vi "Build Filter Command.vi"(8 "error in (no error)":errorcluster, 11 "Filter in":refnum<class "Filter.lvclass">) -> (0 "error out":errorcluster, 2 "Command Words":u16[](array[numeric]) format="%04x")   [LabVIEW 2020, in "BCI-1553 API.lvlib" / "Filter.lvclass"]
doc: "<DO NOT CALL>\n\nThis method is leveraged by the Bus Monitor to produce the raw configuration values for setting up a filter in hardware."
uses:
  Filter.lvclass
  Frames & Messages/TypeDefs/Command Type.ctl
  Filter.lvclass/Filter.ctl
  BCI-1553 API.lvlib
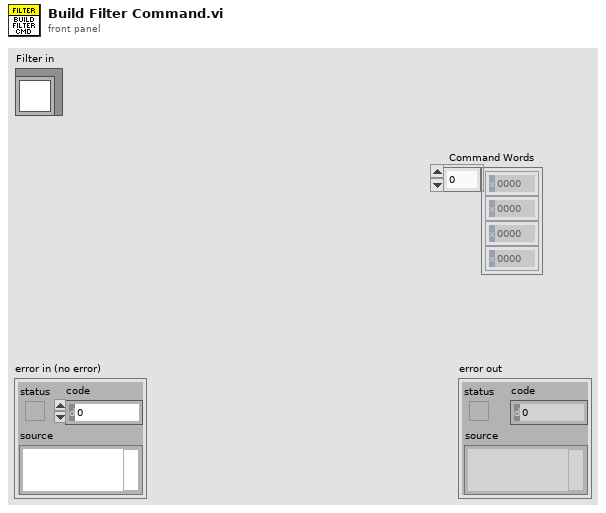
[diagram p1: front panel]
types:
  T1 = typedef "BCI-1553 API.lvlib/Command Type.ctl" = enum16{"Transmit", "Receive"}
  T2 = typedef "BCI-1553 API.lvlib/Command SubAddress.ctl" = enum16{"Mode Code", "1", "2", "3", "4", "5", "6", "7", "8", "9", "10", "11", "12", "13", "14", "15", "16", "17", "18", "19", "20", "21", "22", "23", "24", "25", "26", "27", "28", "29", "30"}
  T3 = typedef "BCI-1553 API.lvlib/Command Terminal Address.ctl" = enum16{"0", "1", "2", "3", "4", "5", "6", "7", "8", "9", "10", "11", "12", "13", "14", "15", "16", "17", "18", "19", "20", "21", "22", "23", "24", "25", "26", "27", "28", "29", "30", "Broadcast"}
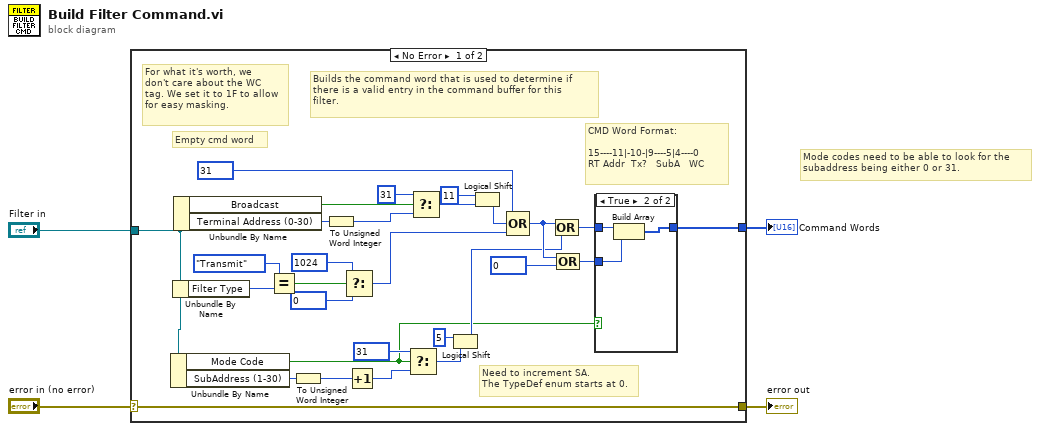
[diagram p0: block diagram]
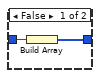
[diagram p2: hidden frame]
diagram:
  # "Mode codes need to be able to look for the\nsubaddress being either 0 or 31."
  n1 = case shown="No Error" "error in (no error)" {
    selector: "error in (no error)" -> [w33 w39]
    tunnel: [w33 w39] -> w3
    tunnel: "Filter in" -> [w32 _]
    tunnel: [w13 _] -> w1
    frame No Error {
      # "Need to increment SA.\nThe TypeDef enum starts at 0."
      # "For what it's worth, we\ndon't care about the WC\ntag. We set it to 1F to allow\nfor easy masking."
      # "CMD Word Format:\n\n15----11|-10-|9----5|4----0\nRT Addr  Tx?   SubA   WC"
      # "Empty cmd word"
      # "Builds the command word that is used to determine if\nthere is a valid entry in the command buffer for this\nfilter."
      n2 = Unbundle By Name(w32) -> ("Mode Code"=w8:bool, "SubAddress (1-30)"=w18:T2)
      n3 = Unbundle By Name(w32) -> ("Filter Type"=w24:T1)
      n4 = Unbundle By Name(w32) -> ("Broadcast"=w30:bool, "Terminal Address (0-30)"=w31:T3)
      n5 = Equal?(x=Command_Type."Transmit", y=w24) -> (x = y?=w22:bool)
      n6 = To Unsigned Word Integer(number=w18) -> (unsigned 16bit integer=w6:u16)
      n7 = To Unsigned Word Integer(number=w31) -> (unsigned 16bit integer=w7:u16)
      n8 = Select(t=u16 1024, s=w22, f=u16 0) -> (s? t:f=w19:u16)
      n9 = Increment(x=w6) -> (x+1=w5:u16)
      n10 = Select(t=u16 31, s=w8, f=w5) -> (s? t:f=w10:u16)
      n11 = Select(t=u16 31, s=w30, f=w7) -> (s? t:f=w27:u16)
      n12 = Logical Shift(y=i16 5, x=w10) -> (x << y=w9:u16)
      n13 = Logical Shift(y=i16 11, x=w27) -> (x << y=w25:u16)
      n14 = Compound Arithmetic op=OR(u16 31, w25, w19) -> (w16:u16)
      n15 = Compound Arithmetic op=OR(w16, w9) -> (w14:u16)
      n16 = Compound Arithmetic op=OR(w16, u16 0) -> (w12:u16)
      n17 = case shown="True" w8 {
        tunnel: w14 -> [w35 w38]
        tunnel: [w34 w37] -> w13
        tunnel: w12 -> [_ w36]
        frame False {
          n18 = Build Array(w35) -> (w34:u16[])
        }
        frame True {
          n19 = Build Array(w38, w36) -> (w37:u16[])
        }
      }
    }
    frame Error {
    }
  }
  "error out" <- w3
  "Command Words" <- w1
